vi "DrawAxes.vi"(3 "Colors":T2={"X Color"=16716800, "Y Color"=1233407, "Z Color"=1441536}, 4 "Axes":T1=[[1.0, 0.0, 0.0, 0.0], [0.0, 1.0, 0.0, 0.0], [0.0, 0.0, 1.0, 0.0], [0.0, 0.0, 0.0, 1.0]], 5 "Stage in":refnum<vi>) -> (2 "Stage out":refnum<vi>)   [LabVIEW 2018]
uses:
  <vilib>/Analysis/Matrix/Datatypes/RealMatrix.ctl
  <vilib>/picture/3D Picture Control/NI_3D Picture Control.lvlib
  <vilib>/Analysis/Matrix/NI_Matrix.lvlib
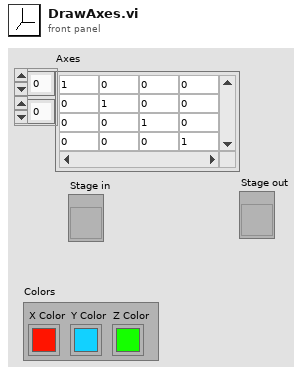
[diagram p1: front panel]
types:
  T1 = typedef "NI_Matrix.lvlib/RealMatrix.ctl" = dbl[][]
  T2 = cluster{"X Color":u32, "Y Color":u32, "Z Color":u32}
  T3 = cluster{"Axes[0]":dbl, "Axes[1]":dbl, "Axes[2]":dbl}
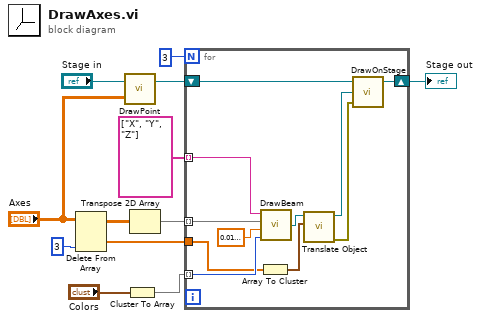
[diagram p0: block diagram]
diagram:
  n1 = Delete From Array(array="Axes", index (col)=3 ("disabled index (col)")) -> (deleted portion=w1:dbl[], array with subset deleted=w6:T1)  [unwired: 2 in]
  n2 = call "DrawPoint.vi"("Start"="Axes", "Stage in"="Stage in") -> ("Stage out"=w8:refnum<vi>)  [unwired: 1 in]
  n3 = Cluster To Array(cluster="Colors") -> (array=w11:u32[])
  n4 = Transpose 2D Array(2D array=w6) -> (transposed array=w3:T1)
  n5 = for {
    N: 3 -> [_]
    tunnel: w3 -> [w16] mode=indexing
    tunnel: w1 -> [w15]
    shift-right: [w13] -> w5
    shift-left: w8 -> [w23]
    tunnel: w11 -> [w21] mode=indexing
    tunnel: string[] ["X", "Y", "Z"] -> [w22] mode=indexing
    n6 = Array To Cluster(array=w15) -> (cluster=w17:T3)
    n7 = call "DrawBeam.vi"("Color"=w21, "Beam radius"=sgl 0.02, "Point"=w16, "Name"=w22) -> ("Beam"=w19:refnum<vi>)  [unwired: 2 in]
    n8 = call <vilib>:"Translate Object.vi"("Translation"=w17, "Scene.Object In"=w19) -> ("error out"=w20:errorcluster, "Scene.Object Out"=w18:refnum<vi>)  [unwired: 8 in]
    n9 = call "DrawOnStage.vi"("error in"=w20, "object in"=w18, "Stage in"=w23) -> ("Stage out"=w13:refnum<vi>)  [unwired: 2 out]
  }
  "Stage out" <- w5
